vi "MainV1.vi"() -> ()   [LabVIEW 2016]
uses:
  Control/StreamCluster.ctl
  Control/GUICluster.ctl
  <vilib>/dex/Stream Element Allocation Mode.ctl
  <vilib>/Platform/TimedLoop/XDataNode/timing_clust.ctl
  <vilib>/Platform/TimedLoop/XDataNode/nitl_modes.ctl
  <vilib>/Platform/TimedLoop/XDataNode/wakeup.ctl
  <vilib>/myRIO/Instrument Drivers/Onboard IO/PWM/typedefs/PWM Reference.ctl
  <vilib>/myRIO/Common/Instrument Driver Framework/Utilities/typedefs/myRIO Generic Hardware Reference.ctl
  <vilib>/myRIO/Common/Instrument Driver Framework/Utilities/typedefs/Hardware Version Enum.ctl
  <vilib>/myRIO/Common/Instrument Driver Framework/Utilities/typedefs/myRIO v1.0 Reference.ctl
  <vilib>/myRIO/Common/Instrument Driver Framework/Utilities/typedefs/Generic FPGA Reference.ctl
  <vilib>/myRIO/Common/Instrument Driver Framework/myRIO v1.0/PWM/typedefs/PWM Channels Enum.ctl
  <vilib>/myRIO/Instrument Drivers/Onboard IO/PWM/typedefs/PWM Configuration.ctl
  <vilib>/userdefined/High Color/nirio_resource_hc.ctl
  <vilib>/myRIO/Instrument Drivers/Onboard IO/AI/typedefs/AI Reference.ctl
  <vilib>/myRIO/Common/Instrument Driver Framework/myRIO v1.0/AI/typedefs/AI Channels List.ctl
  <vilib>/myRIO/Common/Instrument Driver Framework/myRIO v1.0/AI/typedefs/AI Channels Enum.ctl
  <vilib>/myRIO/Common/Instrument Driver Framework/Utilities/typedefs/Analog Scaling Constants List.ctl
  <vilib>/myRIO/Common/Instrument Driver Framework/Utilities/typedefs/Analog Scaling Constants.ctl
  <vilib>/myRIO/Common/Instrument Driver Framework/Utilities/vis/Is FPGA Ref Available.vi
  <vilib>/myRIO/Common/Instrument Driver Framework/myRIO v1.0/AI/vis/myRIO v1.1 Open AI.vi
  <vilib>/myRIO/Instrument Drivers/Onboard IO/AI/vis/Read.vi
  <vilib>/myRIO/Common/Instrument Driver Framework/myRIO v1.0/PWM/vis/myRIO v1.1 Open PWM.vi
  <vilib>/myRIO/Instrument Drivers/Onboard IO/PWM/vis/Set Duty Cycle and Frequency.vi
  <vilib>/myRIO/Common/Instrument Driver Framework/Utilities/vis/Validate Channels.vi
  <vilib>/myRIO/Common/Instrument Driver Framework/myRIO v1.0/AI/vis/myRIO v1.0 Reserve AI.vi
  <vilib>/myRIO/Common/Instrument Driver Framework/myRIO v1.0/PWM/vis/myRIO v1.0 Reserve PWM.vi
  <vilib>/myRIO/Common/Instrument Driver Framework/myRIO v1.0/AI/vis/myRIO v1.0 Build MUX Configuration AI.vi
  <vilib>/myRIO/Common/Instrument Driver Framework/myRIO v1.0/Resource Manager/vis/myRIO v1.0 Reserve Channel List.vi
  <vilib>/myRIO/Common/Instrument Driver Framework/myRIO v1.0/PWM/vis/myRIO v1.0 Build MUX Configuration PWM.vi
  <vilib>/myRIO/Common/Instrument Driver Framework/myRIO v1.0/Resource Manager/vis/myRIO v1.0 Reserve Channel.vi
  <vilib>/myRIO/Common/Instrument Driver Framework/myRIO v1.0/Resource Manager/vis/myRIO v1.0 Unreserve Channel.vi
  <vilib>/myRIO/Common/Instrument Driver Framework/myRIO v1.0/Resource Manager/vis/myRIO v1.0 Create Configuration List.vi
  <vilib>/myRIO/Common/Instrument Driver Framework/myRIO v1.0/Resource Manager/vis/myRIO v1.0 Build Mutex Name.vi
  <vilib>/Utility/VariantDataType/GetNumericInfo.vi
  <vilib>/Utility/error.llb/Error Cluster From Error Code.vi
  <vilib>/myRIO/Common/Instrument Driver Framework/myRIO v1.0/myRIO v1.1 Open.vi
  <vilib>/myRIO/Common/Instrument Driver Framework/Utilities/vis/IO Manager.vi
  <vilib>/myRIO/Common/Instrument Driver Framework/Utilities/vis/Configuration Manager.vi
  <vilib>/myRIO/Common/Instrument Driver Framework/myRIO v1.0/Resource Manager/vis/myRIO v1.0 Configure IO.vi
  <vilib>/myRIO/Common/Instrument Driver Framework/myRIO v1.0/myRIO v1.0 Close.vi
  <vilib>/myRIO/Common/Instrument Driver Framework/myRIO v1.0/PWM/vis/myRIO v1.0 Write PWM.vi
  <vilib>/myRIO/Common/Instrument Driver Framework/myRIO v1.0/AI/vis/myRIO v1.0 Get Scaling Constants AI.vi
  <vilib>/myRIO/Common/Instrument Driver Framework/myRIO v1.0/AI/vis/myRIO v1.0 Read AI.vi
  <vilib>/platform/TimedLoop/XDataNode/XDataNode.xnode
  <vilib>/myRIO/Express VI/Onboard IO/PWM/PWM Express VI.xnode
  <vilib>/myRIO/Instrument Drivers/Onboard IO/PWM/vis/myRIO PWM Open.xnode
  <vilib>/myRIO/Express VI/Onboard IO/AI/AI Express VI.xnode
  <vilib>/myRIO/Instrument Drivers/Onboard IO/AI/vis/myRIO AI Open.xnode
  <vilib>/myRIO/Instrument Drivers/Onboard IO/PWM/PWM.lvlib
  <vilib>/myRIO/Instrument Drivers/Onboard IO/AI/AI.lvlib
  <vilib>/Platform/TimedLoop/XDataNode/XDNodeRunTimeDep.lvlib
panel:
  out "Joule":dbl=-0.1536414641188581
  out "Drehzahl":dbl(knob) scale=0.0..15000.0
  out "GUIInput":T1={"Geschwindigkeitsmultiplikator"=0.0, "Stop"=TRUE, "Start"=FALSE}
  out "output":T2
  out "STOP":bool
  in  "PID Lenkung IR":T3={"proportional gain (Kc)"=0.5, "integral time (Ti, min)"=0.8, "derivative time (Td, min)"=0.002} {"derivative time (Td, min)" format="%.3f"; "integral time (Ti, min)" format="%.3f"; "proportional gain (Kc)" format="%.3f"}
  out "Impulse pro Minute":dbl
  out "counter":dbl=3364.0
  out "Strom":dbl=-0.1536414641188581
  # "Minimum"
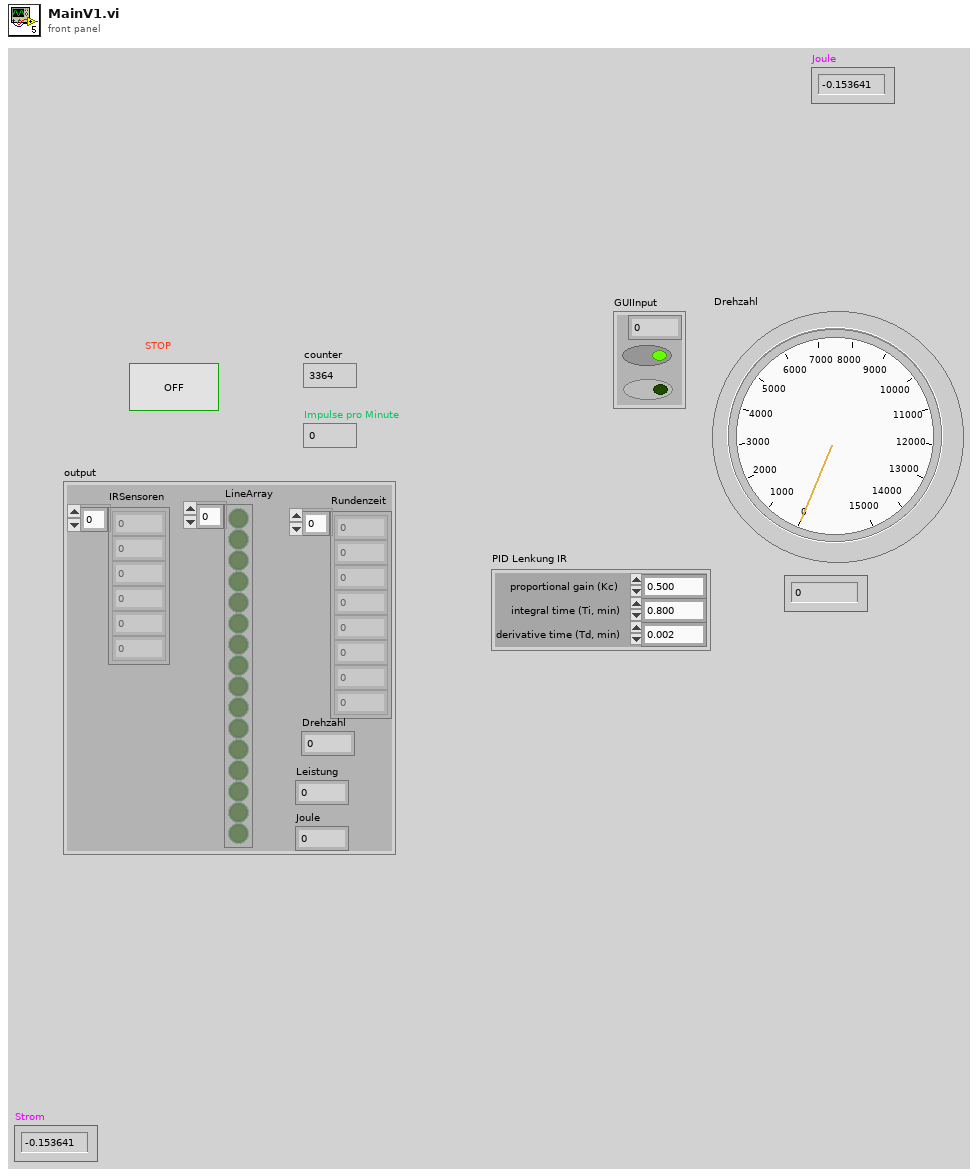
[diagram p1: front panel]
types:
  T1 = typedef "GUICluster.ctl" = cluster{"Geschwindigkeitsmultiplikator":dbl, "Stop":bool, "Start":bool}
  T2 = typedef "StreamCluster.ctl" = cluster{"IRSensoren":dbl[], "LineArray":bool[], "Rundenzeit":dbl[], "Drehzahl":dbl, "Leistung":dbl, "Joule":dbl}
  T3 = cluster{"proportional gain (Kc)":dbl, "integral time (Ti, min)":dbl, "derivative time (Td, min)":dbl}
  T4 = typedef "Stream Element Allocation Mode.ctl" = u32
  T5 = typedef "XDNodeRunTimeDep.lvlib/timing_clust.ctl" = cluster{"Expected End [f-1]":u64, "Actual End [f-1]":u64, "Finished Late? [f-1]":bool, "Expected End [i-1]":u64, "Actual End [i-1]":u64, "Finished Late? [i-1]":bool, "Expected Start [i]":u64, "Actual Start [i]":u64, "Expected Start [f]":u64, "Actual Start [f]":u64, "Source Name":string, "Structure Name":string, "Period":i64, "Deadline":i64, "Offset":i64, "Start":i64, "Priority":i32, "Timeout":i32, "Mode":T6, "Wakeup Reason":T7, "Error":errorcluster, "Source Type":string, "Secondary Source Type":string, "Global End Time":u64, "Global Start Time":u64, "Frame Duration":u64, "Iteration Duration":u64, "Assigned CPU":i32, "I/O Scan Engine Mode":u32}
  T6 = typedef "XDNodeRunTimeDep.lvlib/nitl_modes.ctl" = enum32{"No Change", "Process missed periods, maintain original phase", "Discard missed periods, maintain original phase", "Process missed periods, ignore original phase", "Discard missed periods, ignore original phase"}
  T7 = typedef "XDNodeRunTimeDep.lvlib/wakeup.ctl" = enum32{"Normal", "Aborted", "Asynchronous wakeup", "Timing source error", "Timed loop error", "Timeout"}
  T8 = typedef "AI.lvlib/AI Reference.ctl" = cluster{"myRIO Reference":T9, "AI Channels List":T13, "AI Scaling Constants List":T15}
  T9 = typedef "myRIO Generic Hardware Reference.ctl" = cluster{"myRIO Model":T10, "myRIO Hardware Reference":T11}
  T10 = typedef "Hardware Version Enum.ctl" = enum16{"Unknown", "myRIO-1900", "myRIO-1950", "roboRIO", "NI ELVIS RIO CM"}
  T11 = typedef "myRIO v1.0 Reference.ctl" = cluster{"Generic FPGA Reference":T12, "Allow multiple opens":bool}
  T12 = typedef "Generic FPGA Reference.ctl" = refnum<k20>
  T13 = typedef "AI Channels List.ctl" = T14[]
  T14 = typedef "AI Channels Enum.ctl" = enum16{"Not Connected", "AudioIn/Left", "AudioIn/Right", "C/AI0", "C/AI1", "A/AI0", "A/AI1", "A/AI2", "A/AI3", "B/AI0", "B/AI1", "B/AI2", "B/AI3", "AI/AI0", "AI/AI1", "AI/AI2", "AI/AI3"}
  T15 = typedef "Analog Scaling Constants List.ctl" = T16[]
  T16 = typedef "Analog Scaling Constants.ctl" = cluster{"LSB Weight (Volts)":dbl, "Offset (Volts)":dbl, "Signed?":bool}
  T17 = typedef "nirio_resource_hc.ctl" = tag
  T18 = typedef "PWM.lvlib/PWM Reference.ctl" = cluster{"myRIO Reference":T9, "PWM Channels Enum":T19, "PWM Configuration":T20}
  T19 = typedef "PWM Channels Enum.ctl" = enum16{"Not Connected", "C/PWM0", "C/PWM1", "A/PWM0", "A/PWM1", "A/PWM2", "B/PWM0", "B/PWM1", "B/PWM2", "PWM/PWM0", "PWM/PWM1", "PWM/PWM2", "PWM/PWM3", "PWM/PWM4", "PWM/PWM5", "PWM/PWM6", "PWM/PWM7", "PWM/PWM8", "PWM/PWM9"}
  T20 = typedef "PWM.lvlib/PWM Configuration.ctl" = cluster{"Frequency":dbl, "Duty Cycle":dbl}
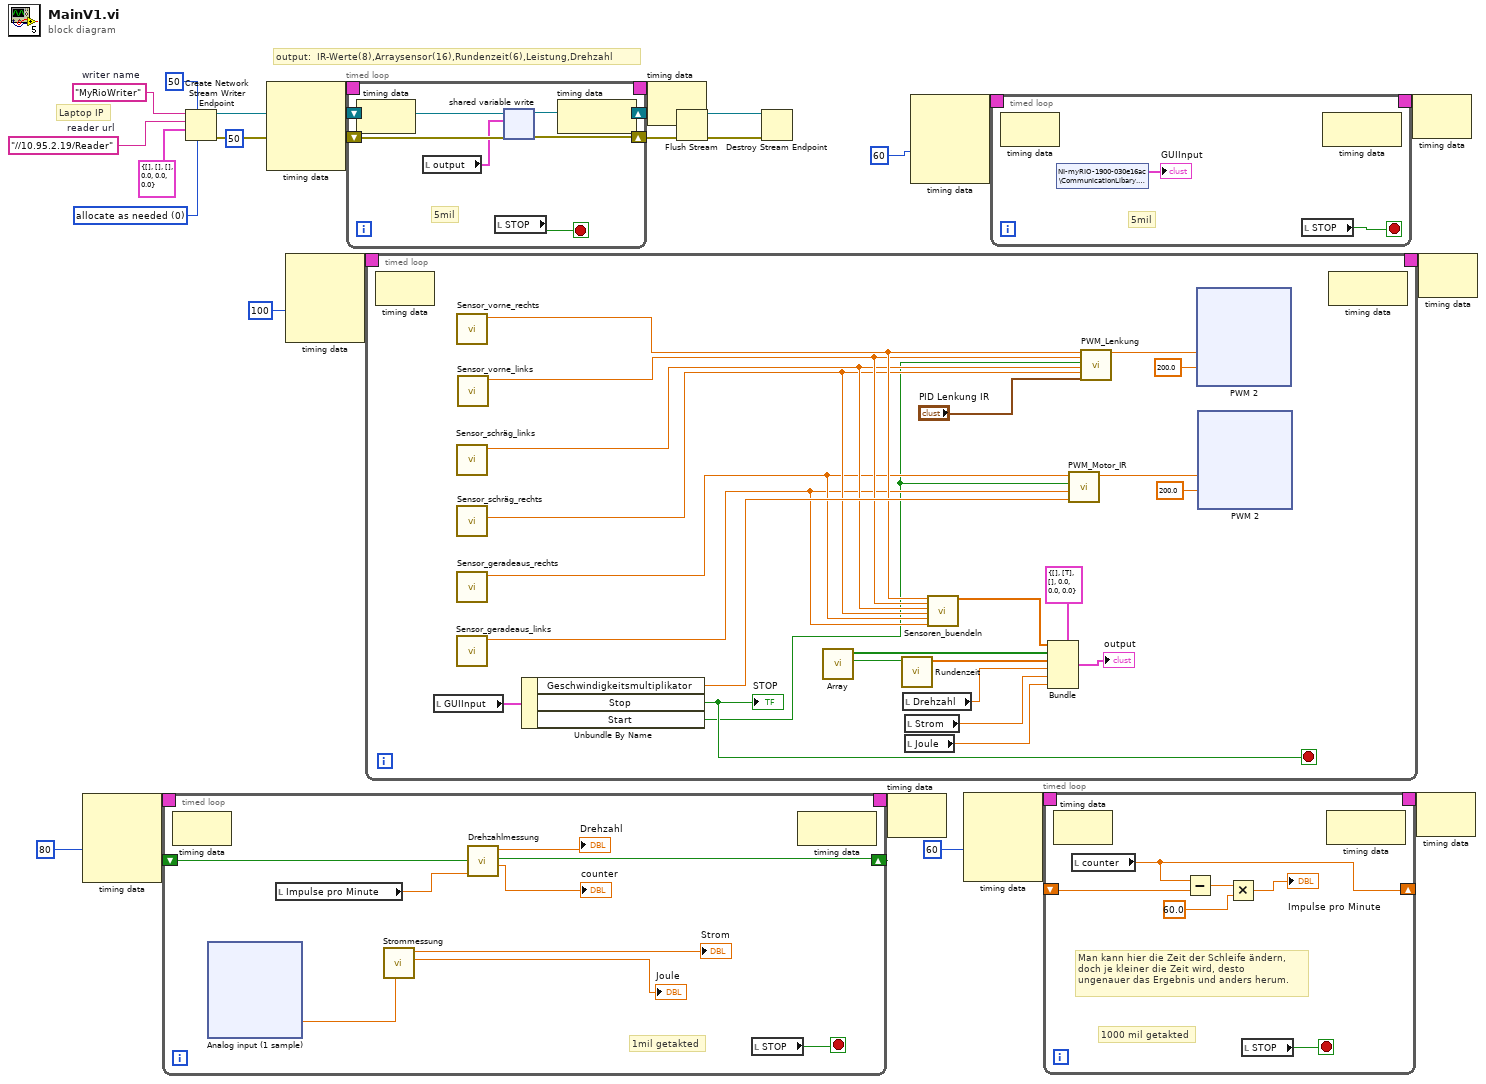
[diagram p0: block diagram]
diagram:
  w16 = T4 0 items=["allocate as needed", "pre-allocate"] ("element allocation mode")
  w25 = "//10.95.2.19/Reader"  # reader url
  w26 = "MyRioWriter"  # writer name
  # "Laptop IP"
  # "output:  IR-Werte(8),Arraysensor(16),Rundenzeit(6),Leistung,Drehzahl"
  n1 = node-c288(80 ("Priority")) -> (w6:T5)  [unwired: 3 in]
  n2 = timed-loop {
    shift-right: [w33] -> _
    shift-left: _ -> [w32]
    timing: w6 -> [_]
    timing-out: [_] -> w5
    stop <- w31 stop-if-true
    # "1mil getakted"
    n3 = node-c288() -> ()  [unwired: 1 in, 1 out]
    n4 = xnode "Analog input (1 sample)"() -> ("C/AI0 (AI0)"=w29:dbl)  [unwired: 1 in, 1 out]
    n5 = local read "Impulse pro Minute"() -> (w35:dbl)
    n6 = call "Strommessung.vi"("Spannung"=w29) -> ("Wattsekunde verbraucht"=→"Joule":dbl, "Strom mit Abweichungen"=→"Strom":dbl)  [unwired: 6 in, 2 out]
    n7 = call "Drehzahlmessung.vi"("Impuls per Minute"=w35, "in"=w32) -> ("counter"=→"counter":dbl, "out"=w33:bool, "Drehzahl"=→"Drehzahl":dbl)  [unwired: 6 in]
    n8 = local read "STOP"() -> (w31:bool)
    n9 = node-c288() -> ()  [unwired: 1 in, 1 out]
  }
  n10 = Create Network Stream Writer Endpoint(6:w16, 7:50 ("writer buffer size"), 9:T2 {"IRSensoren"=[], "LineArray"=[], "Rundenzeit"=[], "Drehzahl"=0.0, "Leistung"=0.0, "Joule"=0.0} ("Cluster"), 10:w25, 11:w26) -> (0:w18:errorcluster, 3:w19:refnum<k21>)  [unwired: 2 in]
  n11 = node-c288(50 ("Priority")) -> (w12:T5)  [unwired: 3 in]
  n12 = node-c288(100 ("Priority")) -> (w15:T5)  [unwired: 3 in]
  n13 = timed-loop {
    shift-right: [w80] -> w21
    shift-left: w19 -> [w78]
    shift-right: [w79] -> w20
    shift-left: w18 -> [w77]
    timing: w12 -> [_]
    timing-out: [_] -> w11
    stop <- w76 stop-if-true
    # "5mil"
    n14 = node-c288() -> ()  [unwired: 1 in, 1 out]
    n15 = local read "output"() -> (w75:T2)
    n16 = local read "STOP"() -> (w76:bool)
    n17 = shared-variable-write(w78, w77, w75) -> (w80:refnum<k21>, w79:errorcluster)  [unwired: 1 in, 1 out]
    n18 = node-c288() -> ()  [unwired: 1 in, 1 out]
  }
  n19 = timed-loop {
    timing: w15 -> [_]
    timing-out: [_] -> w14
    stop <- w100 stop-if-true
    n20 = node-c288() -> ()  [unwired: 1 in, 1 out]
    n21 = local read "GUIInput"() -> (w101:T1)
    n22 = call "Sensor_vorne_rechts.vi"() -> ("Abstand in cm"=w90:dbl)  [unwired: 11 in]
    n23 = call "Sensor_schräg_links.vi"() -> ("Abstand in cm"=w88:dbl)  [unwired: 11 in]
    n24 = call "Sensor_schräg_rechts.vi"() -> ("Abstand in cm"=w87:dbl)  [unwired: 11 in]
    n25 = call "Sensor_geradeaus_rechts.vi"() -> ("Abstand in cm"=w86:dbl)  [unwired: 11 in]
    n26 = call "Sensor_geradeaus_links.vi"() -> ("Abstand in cm"=w85:dbl)  [unwired: 11 in]
    n27 = call "Sensor_vorne_links.vi"() -> ("Abstand in cm"=w89:dbl)  [unwired: 11 in]
    n28 = Unbundle By Name(w101) -> ("Geschwindigkeitsmultiplikator"=w91:dbl, "Stop"=w100:bool, "Start"=w84:bool)
    "STOP" <- w100
    n29 = call "Array.vi"() -> ("Startlinie true"=w92:bool, "array"=w93:bool[])  [unwired: 9 in]
    n30 = call "Rundenzeit.vi"("Startlinie"=w92) -> ("Rundenzeiten"=w98:dbl[])  [unwired: 10 in]
    n31 = local read "Drehzahl"() -> (w97:dbl)
    n32 = local read "Strom"() -> (w96:dbl)
    n33 = local read "Joule"() -> (w83:dbl)
    n34 = call "Sensoren_buendeln.vi"("rechts seite"=w90, "Links seite"=w89, "Links schräg"=w88, "rechts Schräg"=w87, "rechts geradeaus"=w86, "Links Geradeaus"=w85) -> ("SensorArray"=w94:dbl[])  [unwired: 13 in]
    n35 = Bundle(cluster=T2 {"IRSensoren"=[], "LineArray"=[TRUE], "Rundenzeit"=[], "Drehzahl"=0.0, "Leistung"=0.0, "Joule"=0.0} ("Cluster"), "IRSensoren"=w94, "LineArray"=w93, "Rundenzeit"=w98, "Drehzahl"=w97, "Leistung"=w96, "Joule"=w83) -> (→"output":T2)
    n36 = call "PWM_Motor_IR.vi"("Sensorwert"=w86, "Start"=w84, "Sensorwert 2"=w85, "Geschwindigkeit multiplikator"=w91) -> ("PWM Motor"=w103:dbl)  [unwired: 5 in]
    n37 = call "PWM_Lenkung.vi"("vorne rechts"=w90, "vorne links"=w89, "Start"=w84, "Schräg links"=w88, "Schräg rechts"=w87, "PID Werte"="PID Lenkung IR") -> ("PWM Lenkung"=w104:dbl)  [unwired: 13 in]
    n38 = xnode "PWM 2"("Duty Cycle"=w104, "Frequency [Hz]"=200.0 ("y")) -> ()  [unwired: 1 in, 1 out]
    n39 = xnode "PWM 2"("Duty Cycle"=w103, "Frequency [Hz]"=200.0) -> ()  [unwired: 1 in, 1 out]
    n40 = node-c288() -> ()  [unwired: 1 in, 1 out]
  }
  n41 = node-c288(w11) -> ()  [unwired: 1 out]
  n42 = Flush Stream(8:w20, 11:w21) -> (0:w23:errorcluster, 3:w22:refnum<k21>)  [unwired: 2 in, 1 out]
  n43 = Destroy Stream Endpoint(8:w23, 11:w22) -> ()  [unwired: 1 out]
  n44 = node-c288(w5) -> ()  [unwired: 1 out]
  n45 = node-c288(60 ("Priority")) -> (w9:T5)  [unwired: 3 in]
  n46 = node-c288(60 ("Priority")) -> (w3:T5)  [unwired: 3 in]
  n47 = timed-loop {
    timing: w9 -> [_]
    timing-out: [_] -> w8
    stop <- w179 stop-if-true
    # "5mil"
    n48 = node-c288() -> ()  [unwired: 1 in, 1 out]
    n49 = shared-variable "NI-myRIO-1900-030e16ac\\CommunicationLibary.lvlib\\GUIInput"() -> (→"GUIInput":T1)  [unwired: 1 in, 1 out]
    n50 = local read "STOP"() -> (w179:bool)
    n51 = node-c288() -> ()  [unwired: 1 in, 1 out]
  }
  n52 = timed-loop {
    shift-right: [w188] -> _
    shift-left: _ -> [w187]
    timing: w3 -> [_]
    timing-out: [_] -> w2
    stop <- w183 stop-if-true
    # "1000 mil getakted"
    # "Man kann hier die Zeit der Schleife ändern, \ndoch je kleiner die Zeit wird, desto\nungenauer das Ergebnis und anders herum."
    n53 = node-c288() -> ()  [unwired: 1 in, 1 out]
    n54 = local read "counter"() -> (w188:dbl)
    n55 = Subtract(x=w188, y=w187) -> (x-y=w185:dbl)
    n56 = Multiply(x=w185, y=60.0) -> (x*y=→"Impulse pro Minute":dbl)
    n57 = local read "STOP"() -> (w183:bool)
    n58 = node-c288() -> ()  [unwired: 1 in, 1 out]
  }
  n59 = node-c288(w8) -> ()  [unwired: 1 out]
  n60 = node-c288(w2) -> ()  [unwired: 1 out]
  n61 = node-c288(w14) -> ()  [unwired: 1 out]
